vi "raptor_send_images.vi"(8 "error in (no error)":errorcluster, 9 "Time Stamp":timestamp, 10 "Image Channel 2":T1, 11 "Image Channel 1":T1) -> (0 "error out":errorcluster)   [LabVIEW 2016]
doc: "Raptor: Send OCT B-scan and (optionally) fluorescence line for processing."
uses:
  <vilib>/vision/Image Controls.llb/IMAQ Image.ctl
  typedef/raptor_image.ctl
  globals/Channel 1 Image Ring.vi
  globals/Channel 2 Image Ring.vi
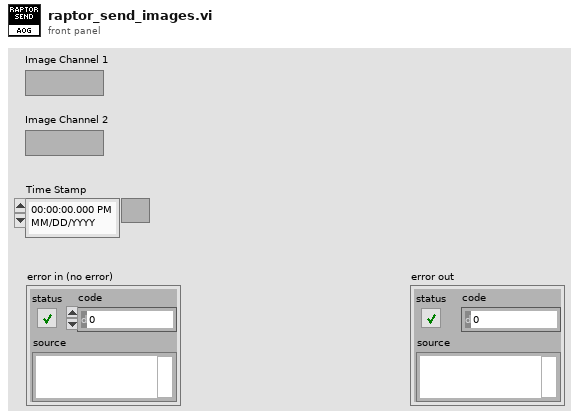
[diagram p1: front panel]
types:
  T1 = typedef "IMAQ Image.ctl" = refnum<image>
  T2 = typedef "raptor_image.ctl" = cluster{"Data":variant, "Image":T1}
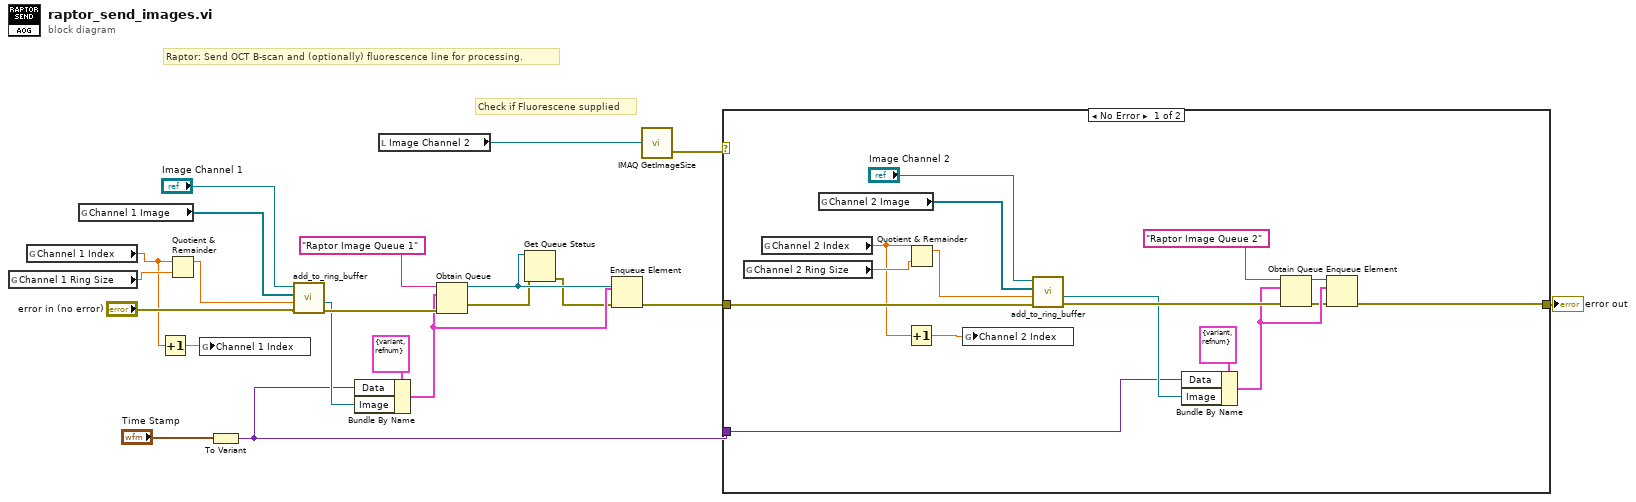
[diagram p0: block diagram]
diagram:
  # "Raptor: Send OCT B-scan and (optionally) fluorescence line for processing."
  # "Check if Fluorescene supplied"
  n1 = global read "Channel 1 Image Ring.vi" "Channel 1 Ring Size"() -> (w21:dbl)
  n2 = global read "Channel 1 Image Ring.vi" "Channel 1 Index"() -> (w9:dbl)
  n3 = global read "Channel 1 Image Ring.vi" "Channel 1 Image"() -> (w20:T1[])
  n4 = Increment(x=w9) -> (x+1=w8:dbl)
  n5 = Quotient & Remainder(x=w9, y=w21) -> (x-y*floor(x/y)=w19:dbl)  [unwired: 1 out]
  n6 = global write "Channel 1 Image Ring.vi" "Channel 1 Index"(w8) -> ()
  n7 = To Variant(anything="Time Stamp") -> (Variant=w10:variant)
  n8 = call "add_to_ring_buffer.vi"("error in"="error in (no error)", "Buffer Position"=w19, "Ring Buffer"=w20, "Image"="Image Channel 1") -> ("error out"=w16:errorcluster, "Buffer Image Out"=w12:T1)  [unwired: 4 in, 2 out]
  n9 = Bundle By Name(cluster=T2 {"Data"=variant, "Image"=refnum} ("Cluster"), "Data"=w10, "Image"=w12) -> (w7:T2)
  n10 = local read "Image Channel 2"() -> (w6:T1)
  n11 = Obtain Queue(name (unnamed)="Raptor Image Queue 1", element data type=w7, error in (no error)=w16) -> (queue out=w4:refnum<queue>, error out=w3:errorcluster)  [unwired: 2 in, 1 out]
  n12 = Get Queue Status(queue=w4, error in (no error)=w3) -> (error out=w2:errorcluster)  [unwired: 1 in, 7 out]
  n13 = Enqueue Element(queue=w4, element=w7, error in (no error)=w2) -> (error out=w1:errorcluster)  [unwired: 1 in, 2 out]
  n14 = call "IMAQ GetImageSize"("Image"=w6) -> ("error out"=w5:errorcluster)  [unwired: 3 in, 2 out]
  n15 = case shown="No Error" w5 {
    tunnel: w1 -> [w33 w38]
    tunnel: [w22 w38] -> w14
    tunnel: w10 -> [w28 _]
    frame No Error {
      n16 = global read "Channel 2 Image Ring.vi" "Channel 2 Ring Size"() -> (w35:dbl)
      n17 = global read "Channel 2 Image Ring.vi" "Channel 2 Index"() -> (w27:dbl)
      n18 = global read "Channel 2 Image Ring.vi" "Channel 2 Image"() -> (w36:T1[])
      n19 = Increment(x=w27) -> (x+1=w26:dbl)
      n20 = Quotient & Remainder(x=w27, y=w35) -> (x-y*floor(x/y)=w37:dbl)  [unwired: 1 out]
      n21 = global write "Channel 2 Image Ring.vi" "Channel 2 Index"(w26) -> ()
      n22 = call "add_to_ring_buffer.vi"("error in"=w33, "Buffer Position"=w37, "Ring Buffer"=w36, "Image"="Image Channel 2") -> ("error out"=w31:errorcluster, "Buffer Image Out"=w29:T1)  [unwired: 4 in, 2 out]
      n23 = Bundle By Name(cluster=T2 {"Data"=variant, "Image"=refnum} ("Cluster"), "Data"=w28, "Image"=w29) -> (w24:T2)
      n24 = Obtain Queue(name (unnamed)="Raptor Image Queue 2", element data type=w24, error in (no error)=w31) -> (queue out=w25:refnum<queue>, error out=w23:errorcluster)  [unwired: 2 in, 1 out]
      n25 = Enqueue Element(queue=w25, element=w24, error in (no error)=w23) -> (error out=w22:errorcluster)  [unwired: 1 in, 2 out]
    }
    frame Error {
    }
  }
  "error out" <- w14
